vi "Get Column Headers.vi"(8 "error in (no error)":errorcluster, 11 "List Box View Model in":refnum<class "List Box Event Log View Model.lvclass">) -> (0 "error out":errorcluster, 2 "Header Strings":string[](array[string]), 3 "List Box View Model out":refnum<class "List Box Event Log View Model.lvclass">)   [LabVIEW 2020, in "List Box Event Log View Model.lvclass"]
uses:
  List Box Event Log View Model.lvclass
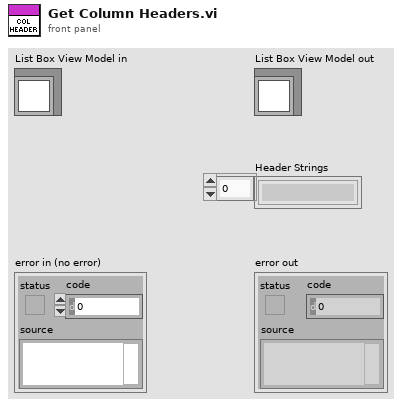
[diagram p1: front panel]
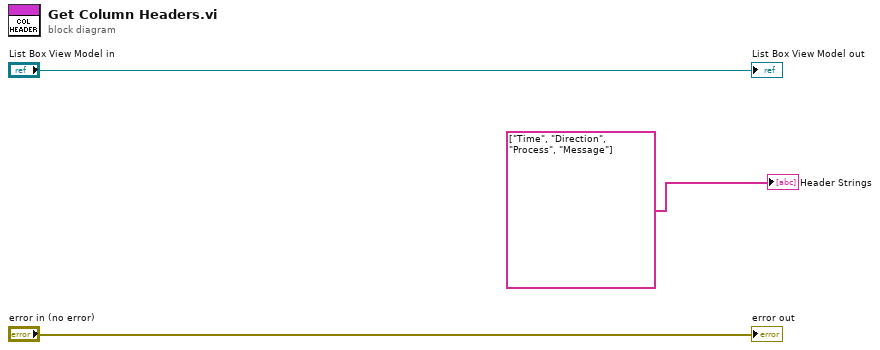
[diagram p0: block diagram]
diagram:
  "error out" <- "error in (no error)"
  "List Box View Model out" <- "List Box View Model in"
  "Header Strings" <- string[] ["Time", "Direction", "Process", "Message"] ("Array")
